vi "Get Absolute Date Time.vi"(0 "VISA resource name":refnum<visa-resource-name>, 11 "error in (no error)":errorcluster) -> (3 "Hour":i32, 4 "VISA resource name out":refnum<visa-resource-name>, 6 "Year":i32, 8 "Month":i32, 10 "Day":i32, 13 "Second":i32, 14 "Minute":i32, 15 "error out":errorcluster)   [LabVIEW 2018, in "Keithley DMM7512.lvlib"]
doc: "This gets the System Time."
uses:
  <instrlib>/Keithley DMM7512/Keithley DMM7512.lvlib
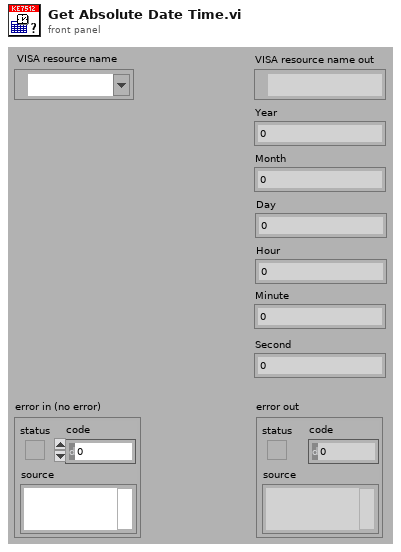
[diagram p1: front panel]
types:
  T1 = cluster{"[0]":string, "[1]":string, "[2]":string, "[3]":string, "[4]":string, "[5]":string, "[6]":string, "[7]":string, "[8]":string}
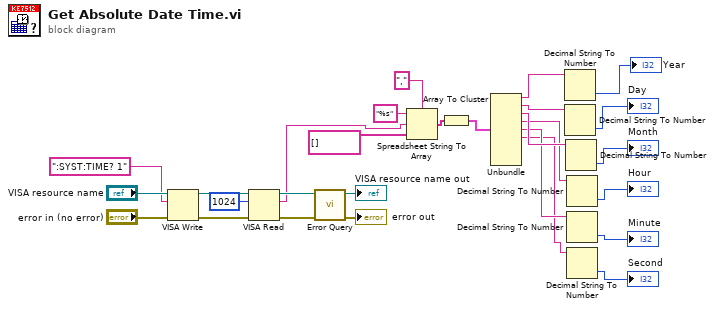
[diagram p0: block diagram]
diagram:
  n1 = VISA Write(VISA resource name="VISA resource name", write buffer=":SYST:TIME? 1", error in (no error)="error in (no error)") -> (VISA resource name out=w27:refnum<visa-resource-name>, error out=w28:errorcluster)  [unwired: 1 out]
  n2 = VISA Read(VISA resource name=w27, byte count=u32 1024, error in (no error)=w28) -> (VISA resource name out=w21:refnum<visa-resource-name>, read buffer=w18:string, error out=w20:errorcluster)  [unwired: 1 out]
  n3 = call <instrlib>:"Error Query.vi"("error in (no error)"=w20, "VISA resource name"=w21) -> ("error out"=→"error out":errorcluster, "VISA resource name out"=→"VISA resource name out":refnum<visa-resource-name>)  [unwired: 8 out]
  n4 = Spreadsheet String To Array(delimiter (Tab)=",", format string="%s", spreadsheet string=w18, array type (2D Dbl)=string[] []) -> (array=w14:string[])
  n5 = Array To Cluster(array=w14) -> (cluster=w13:T1)
  n6 = Unbundle(w13) -> ("[0]"=w11:string, "[1]"=w10:string, "[2]"=w9:string, "[3]"=w8:string, "[4]"=w7:string, "[5]"=w6:string)  [unwired: 3 out]
  n7 = Decimal String To Number(string=w11) -> (number=→"Year":i32)  [unwired: 2 in, 1 out]
  n8 = Decimal String To Number(string=w10) -> (number=→"Day":i32)  [unwired: 2 in, 1 out]
  n9 = Decimal String To Number(string=w9) -> (number=→"Month":i32)  [unwired: 2 in, 1 out]
  n10 = Decimal String To Number(string=w8) -> (number=→"Hour":i32)  [unwired: 2 in, 1 out]
  n11 = Decimal String To Number(string=w7) -> (number=→"Minute":i32)  [unwired: 2 in, 1 out]
  n12 = Decimal String To Number(string=w6) -> (number=→"Second":i32)  [unwired: 2 in, 1 out]
